vi "comparison.vi"(3 "error in (no error)":errorcluster, 4 "new Variable Cluster":T1, 5 "original Variable Cluster":T1) -> (0 "error out":errorcluster, 1 "Variable Cluster":T1, 2 "change":bool)   [LabVIEW 2012, in "HGF_SV.lvlib" / "HGF_SVMonitor.lvclass"]
doc: "Compare variables for\ntrue: timestamp change or\nfalse: variant data (to string) change"
uses:
  HGF_SVMonitor.lvclass
  HGF_BaseClasses/HGF_NetworkVisitor/HGF_NetworkVisitor.lvclass
  HGF_BaseClasses/HGF_TriggeredEvent/HGF_TriggeredEvent.lvclass
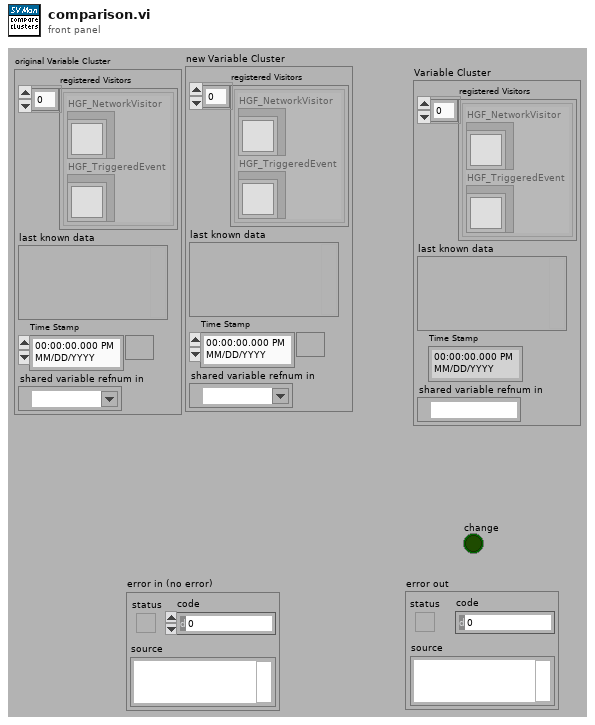
[diagram p1: front panel]
types:
  T1 = cluster{"registered Visitors":cluster{"HGF_NetworkVisitor":refnum<class "HGF_NetworkVisitor.lvclass">, "HGF_TriggeredEvent":refnum<class "HGF_TriggeredEvent.lvclass">}[], "last known data":variant, "Time Stamp":timestamp, "shared variable refnum in":refnum<k21>}
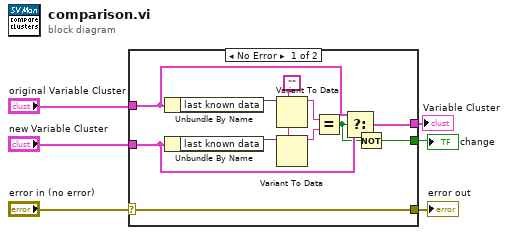
[diagram p0: block diagram]
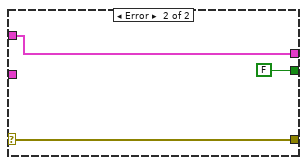
[diagram p2: hidden frame]
diagram:
  n1 = case shown="No Error" "error in (no error)" {
    selector: "error in (no error)" -> [w13 w18]
    tunnel: "original Variable Cluster" -> [w17 w20]
    tunnel: "new Variable Cluster" -> [w16 _]
    tunnel: [w15 w20] -> w1
    tunnel: [w14 FALSE] -> w5
    tunnel: [w13 w18] -> w4
    frame No Error {
      w10 = ""
      n2 = Unbundle By Name(w17) -> ("last known data"=w12:variant)
      n3 = Unbundle By Name(w16) -> ("last known data"=w11:variant)
      n4 = Variant To Data(type=w10, Variant=w12) -> (data=w9:string)  [unwired: 1 in, 1 out]
      n5 = Variant To Data(type=w10, Variant=w11) -> (data=w8:string)  [unwired: 1 in, 1 out]
      n6 = Equal?(x=w9, y=w8) -> (x = y?=w7:bool)
      n7 = Select(t=w17, s=w7, f=w16) -> (s? t:f=w15:T1)
      n8 = Not(x=w7) -> (.not. x?=w14:bool)
    }
    frame Error {
    }
  }
  "change" <- w5
  "error out" <- w4
  "Variable Cluster" <- w1
